vi "Setup.vi"(11 "Template Event in":refnum<class "Template Event.lvclass">) -> (3 "Template Event out":refnum<class "Template Event.lvclass">)   [LabVIEW 2021, in "Template Event.lvlib" / "Template Event.lvclass"]
uses:
  Template Event.lvclass
  Template Event.lvclass/Template Event.ctl
  <vilib>/Nathan Davis/jettl/jettl/Event/Event.lvclass
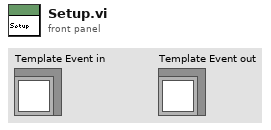
[diagram p1: front panel]
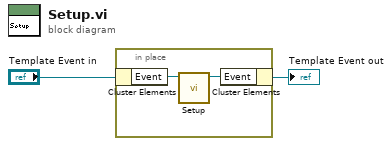
[diagram p0: block diagram]
diagram:
  n1 = in-place {
    n2 = in-place-cluster #1("Template Event in") -> ("Event"=w4:refnum<class "Event.lvclass">)
    n3 = call-dynamic "Setup.vi"("jettl Msg Setup in"=w4) -> ("jettl Msg Setup out"=w3:refnum<class "Event.lvclass">)  [unwired: 10 in]
    n4 = in-place-cluster #1("Event"=w3) -> (→"Template Event out":refnum<class "Template Event.lvclass">)
  }
